vi "relative access path.vi"(11 "Oauth2.Harvest":refnum<class "Oauth2.Harvest.lvclass">) -> (1 "Token Access Path":string, 2 "Authorization Path":string)   [LabVIEW 2020, in "Oauth2.Harvest.lvclass"]
uses:
  Oauth2.Harvest.lvclass
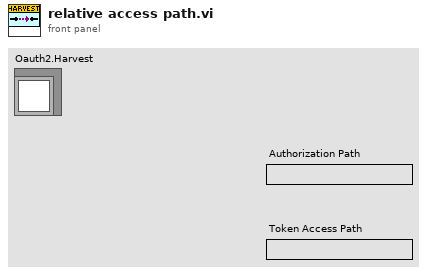
[diagram p1: front panel]
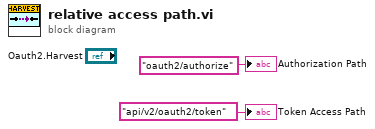
[diagram p0: block diagram]
diagram:
  "Authorization Path" <- "oauth2/authorize" ("Authorization Path")
  "Token Access Path" <- "api/v2/oauth2/token" ("Authorization Path")
